vi "EIP Read Tags.vi"(6 "Tag Data":T3[](array[typedef]) {"Device Reference" format="%.0x"}, 7 "Device Settings":T2, 8 "error in":errorcluster, 9 "Session In":T1, 10 "Device Outputs In":dbl[](array[numeric]), 11 "Device Outputs FIFO":refnum<k33>) -> (0 "error out":errorcluster, 1 "Session Out":T1, 2 "Device Outputs Out":dbl[](array[numeric]))   [LabVIEW 2011, in "Ethernet IP Custom Device Custom Device.lvlib"]
uses:
  Ethernet IP Custom Device Custom Device.lvlib
  EIP Tag Information.ctl
  <vilib>/NI Veristand/Custom Device API/Custom Device Item Info.ctl
  <vilib>/NI Veristand/Custom Device API/Custom Device Item Ref.ctl
  L5K Data Types.ctl
  EIP Device Settings.ctl
  <vilib>/ethernetip/ethernetip.llb/ethernetip.ctl
  <vilib>/ethernetip/ethernetip.llb/EthernetIP Tag Read INT.vi
  <vilib>/ethernetip/ethernetip.llb/EthernetIP Tag Read DINT.vi
  <vilib>/ethernetip/ethernetip.llb/EthernetIP Tag Read REAL.vi
  <vilib>/ethernetip/ethernetip.llb/EthernetIP Tag Read BOOL.vi
  <vilib>/ethernetip/ethernetip.llb/EthernetIP Tag Read SINT.vi
  <vilib>/ethernetip/ethernetip.lvlib
  <vilib>/NI Veristand/Custom Device API/Custom Device API.lvlib
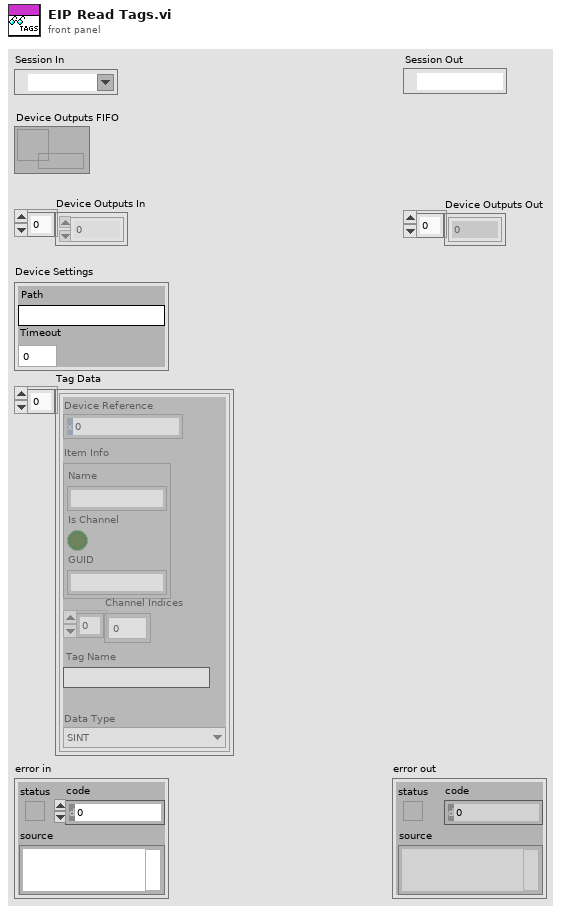
[diagram p1: front panel]
types:
  T1 = typedef "ethernetip.lvlib/ethernetip.ctl" = refnum<k21>
  T2 = typedef "Ethernet IP Custom Device Custom Device.lvlib/EIP Device Settings.ctl" = cluster{"Path":string, "Timeout":i32}
  T3 = typedef "Ethernet IP Custom Device Custom Device.lvlib/EIP Tag Information.ctl" = cluster{"Item Info":T4, "Device Reference":T5, "Channel Indices":i32[], "Tag Name":string, "Data Type":T6}
  T4 = typedef "Custom Device API.lvlib/Custom Device Item Info.ctl" = cluster{"Name":string, "Is Channel":bool, "GUID":string}
  T5 = typedef "Custom Device API.lvlib/Custom Device Item Ref.ctl" = u64
  T6 = typedef "Ethernet IP Custom Device Custom Device.lvlib/L5K Data Types.ctl" = enum16{"SINT", "INT", "DINT", "REAL", "BOOL"}
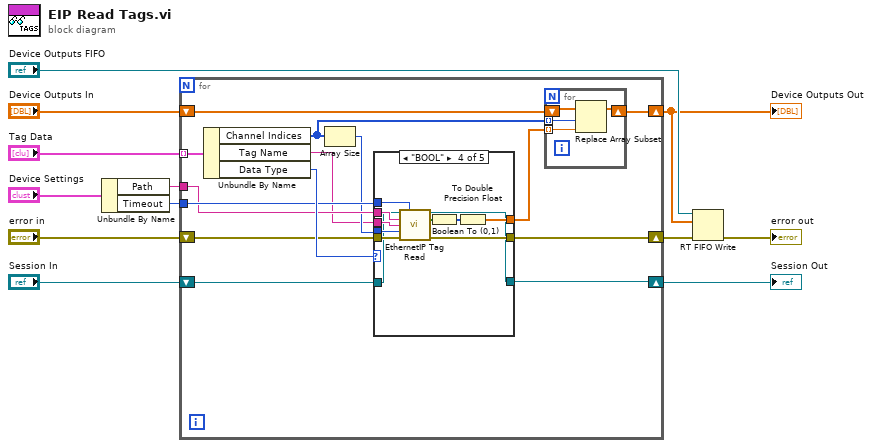
[diagram p0: block diagram]
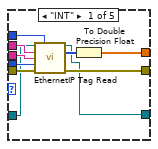
[diagram p2: hidden frame]
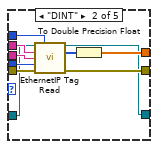
[diagram p3: hidden frame]
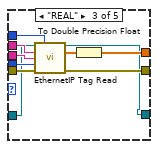
[diagram p4: hidden frame]
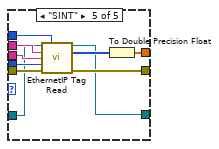
[diagram p5: hidden frame]
diagram:
  n1 = Unbundle By Name("Device Settings") -> ("Path"=w8:string, "Timeout"=w7:i32)
  n2 = for {
    shift-right: [w17] -> w3
    shift-left: "Device Outputs In" -> [w18]
    tunnel: "Tag Data" -> [w26] mode=indexing
    shift-right: [w23] -> w5
    shift-left: "error in" -> [w24]
    tunnel: w8 -> [w21]
    tunnel: w7 -> [w22]
    shift-right: [w13] -> w1
    shift-left: "Session In" -> [w14]
    n3 = Unbundle By Name(w26) -> ("Channel Indices"=w16:i32[], "Tag Name"=w19:string, "Data Type"=w25:T6)
    n4 = Array Size(array=w16) -> (size(s)=w20:i32)
    n5 = case shown="\"BOOL\"" w25 {
      tunnel: w20 -> [w36 w46 w56 w68 w78]
      tunnel: [w39 w49 w59 w70 w73] -> w23
      tunnel: [w38 w48 w58 w63 w80] -> w15
      tunnel: w21 -> [w37 w47 w57 w69 w79]
      tunnel: w19 -> [w35 w45 w55 w67 w75]
      tunnel: w24 -> [w34 w44 w54 w66 w77]
      tunnel: w22 -> [w33 w43 w53 w65 w76]
      tunnel: w14 -> [w31 w42 w52 w61 w74]
      tunnel: [w32 w41 w51 w62 w72] -> w13
      frame "INT" {
        n6 = call-poly <vilib>:"EthernetIP Tag Read.vi"("Session in"=w31, "Timeout (ms)"=w33, "Network Path"=w37, "Tag Name"=w35, "Number of Elements"=w36, "error in"=w34) -> ("Session out"=w32:T1, "Data"=w40:i16[], "error out"=w39:errorcluster)  [unwired: 7 in]
        n7 = To Double Precision Float(number=w40) -> (double precision float=w38:dbl[])
      }
      frame "DINT" {
        n8 = call-poly <vilib>:"EthernetIP Tag Read.vi"("Session in"=w42, "Timeout (ms)"=w43, "Network Path"=w47, "Tag Name"=w45, "Number of Elements"=w46, "error in"=w44) -> ("Session out"=w41:T1, "Data"=w50:i32[], "error out"=w49:errorcluster)  [unwired: 7 in]
        n9 = To Double Precision Float(number=w50) -> (double precision float=w48:dbl[])
      }
      frame "REAL" {
        n10 = call-poly <vilib>:"EthernetIP Tag Read.vi"("Session in"=w52, "Timeout (ms)"=w53, "Network Path"=w57, "Tag Name"=w55, "Number of Elements"=w56, "error in"=w54) -> ("Session out"=w51:T1, "Data"=w60:sgl[], "error out"=w59:errorcluster)  [unwired: 7 in]
        n11 = To Double Precision Float(number=w60) -> (double precision float=w58:dbl[])
      }
      frame "BOOL" {
        n12 = call-poly <vilib>:"EthernetIP Tag Read.vi"("Session in"=w61, "Timeout (ms)"=w65, "Network Path"=w69, "Tag Name"=w67, "Number of Elements"=w68, "error in"=w66) -> ("Session out"=w62:T1, "Data"=w71:bool[], "error out"=w70:errorcluster)  [unwired: 7 in]
        n13 = Boolean To (0,1)(Boolean=w71) -> (0, 1=w64:i16[])
        n14 = To Double Precision Float(number=w64) -> (double precision float=w63:dbl[])
      }
      frame "SINT" {
        n15 = call-poly <vilib>:"EthernetIP Tag Read.vi"("Session in"=w74, "Timeout (ms)"=w76, "Network Path"=w79, "Tag Name"=w75, "Number of Elements"=w78, "error in"=w77) -> ("Session out"=w72:T1, "Data"=w81:i8[], "error out"=w73:errorcluster)  [unwired: 7 in]
        n16 = To Double Precision Float(number=w81) -> (double precision float=w80:dbl[])
      }
    }
    n17 = for {
      tunnel: w15 -> [w28] mode=indexing
      tunnel: w16 -> [w29] mode=indexing
      shift-right: [w27] -> w17
      shift-left: w18 -> [w30]
      n18 = Replace Array Subset(array=w30, new element=w28, index=w29) -> (w27:dbl[])
    }
  }
  "Device Outputs Out" <- w3
  "Session Out" <- w1
  n19 = RT FIFO Write(0:"Device Outputs FIFO", 1:w3, 3:w5) -> (11:→"error out":errorcluster)  [unwired: 1 in, 4 out]
